vi "TagDB dbChanged.vi"(8 "error in (no error)":errorcluster, 11 "DB Ref":refnum<k1>) -> (0 "error in (no error) (dup)":errorcluster, 2 "changed?":bool, 3 "DB Ref (dup)":refnum<k1>)   [LabVIEW 2017, in "TagDB.lvlib"]
uses:
  TagDB.lvlib
  Error/_[error50000]Invalid DB REF.vi
  DataAccess/TagDB Ref to DVR.vi
  Error/_Build Error Cluster.vi
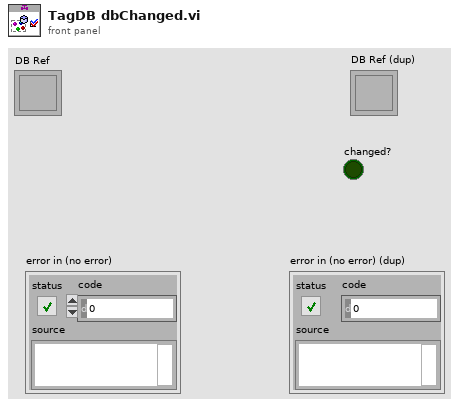
[diagram p1: front panel]
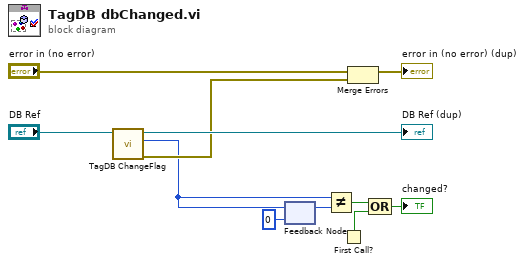
[diagram p0: block diagram]
diagram:
  n1 = call "TagDB ChangeFlag.vi"("DB Ref"="DB Ref") -> ("error in (no error) (dup)"=w7:errorcluster, "Global Change Timestamp"=w2:u64, "DB Ref (dup)"=→"DB Ref (dup)":refnum<k1>)  [unwired: 7 in, 1 out]
  n2 = feedback-in #1(w2) -> ()
  n3 = feedback #1(u64 0 ("Global Change Timestamp")) -> (w3:u64)
  n4 = Not Equal?(x=w2, y=w3) -> (x != y?=w5:bool)
  n5 = First Call?() -> (First Call?: T/F=w6:bool)
  n6 = Merge Errors("error in (no error)", w7) -> (→"error in (no error) (dup)":errorcluster)
  n7 = Compound Arithmetic op=OR(w5, w6) -> (→"changed?":bool)
